vi "ErrorHandler.vi"(5 "user message (\"\")":string, 6 "exception code (0=no exception)":i32, 7 "error description (\"\")":string, 8 "error in (no error)":errorcluster, 11 "error code (0)":i32 format="%0.0f") -> (0 "error out":errorcluster, 2 "Error info":T1)   [LabVIEW 2013, in "SMP.lvclass"]
doc: "Produces an error cluster with a source string that contains all error details in a JSON object. The elements of the JSON object are: Code, Source, Description, Call chain, User message.\n\nThe Description contains the actual/possible cause of the error. This is the standard description that Labview shows when debugging. The \"error in\" input has first priority, so if an error is present here it will be output in \"error out\" with the formatted source string.\n\n<b>error code: </b>If \"error in\" has no error then a custom error will be generated if this code is not 0. The source string of the custom error will have this code, the description from the \"error description\" input, the user message from the \"user message\" input and the call chain up to the VI calling this Error Handler.\n\n<b>error description: </b>The description for the custom error, to be included in the JSON object held in the error source string.\n\n<b>user message: </b>The user message associated with the custom error, to be included in the JSON object held in the error source string.\n\n<b>exception code: </b> Specifies a particular error code to be ignored. This option only works for errors received via the \"error in\" input. If this code is received, the handler will clear the error.\n\n<b>Error info: </b>A cluster containing all error info. This is provided for convenience. It contains exactly the same information as the JSON object held in the error source string."
uses:
  SMP.lvclass
  70a9a6cd-0d05-4d49-a097-5f9bfbe52c2b.vi
  1c7ce2ab-558f-46e0-889c-9a5a86a7245e.vi
  df1b85dd-af5c-4eb8-b3ac-6a4bf91d912d.vi
  cf7a518e-8a90-4b9b-b245-fd60522d3528.vi
  <vilib>/JDP Science/JSONtext/JSONtext.lvlib
  8e39f65f-b52b-460e-aed2-aa7242cb256d.vi
  9ede7785-e4b7-4a2b-ad65-c3c71cf36ef6.vi
  5dddf332-14d7-45ee-9639-52c0eabf6bef.vi
  e595dffb-a454-4284-baeb-2219d1b7dc43.vi
  e26eb3da-07b3-4e20-90df-f977e2e68984.vi
  <vilib>/Utility/error.llb/DialogType.ctl
  debc1eb8-1280-4e15-8515-044490ebb883.vi
  e2486d55-95a2-4599-8c71-563c50abe2ef.vi
  3d1d037f-df6a-40d9-93cf-b9c414a2865f.vi
  7ecf2d71-b2a8-4580-9142-73392cecd242.vi
  1f3aeea1-64a9-4bcd-a0b4-ffb7e781f43c.vi
  b1e9468c-6006-4e50-9a64-d51c3021ee35.vi
  89762134-3b04-4251-8c1b-3ad095ef116d.vi
  12af56b0-901a-41e5-9ea6-8feb9238e45a.vi
  6ee8f00d-676c-48f5-90a6-41a3b84b36f5.vi
  105fa579-688c-41c6-a4d2-67f13b08f2ab.vi
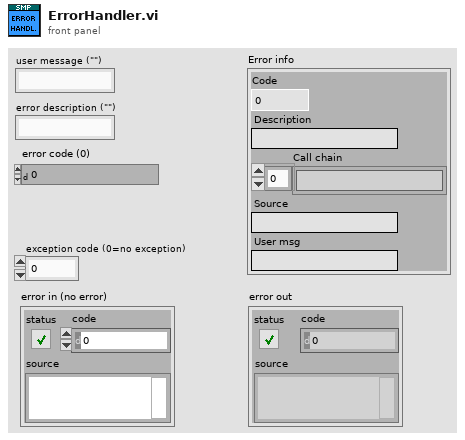
[diagram p1: front panel]
types:
  T1 = cluster{"Code":i32, "Description":string, "Call chain":string[], "Source":string, "User msg":string}
  T2 = typedef "JSONtext.lvlib/JSON Value Type.ctl" = enum16{"Not a JSON Value", "JSON Object", "JSON Array", "String", "Number", "true", "false", "null"}
  T3 = typedef "DialogType.ctl" = u16
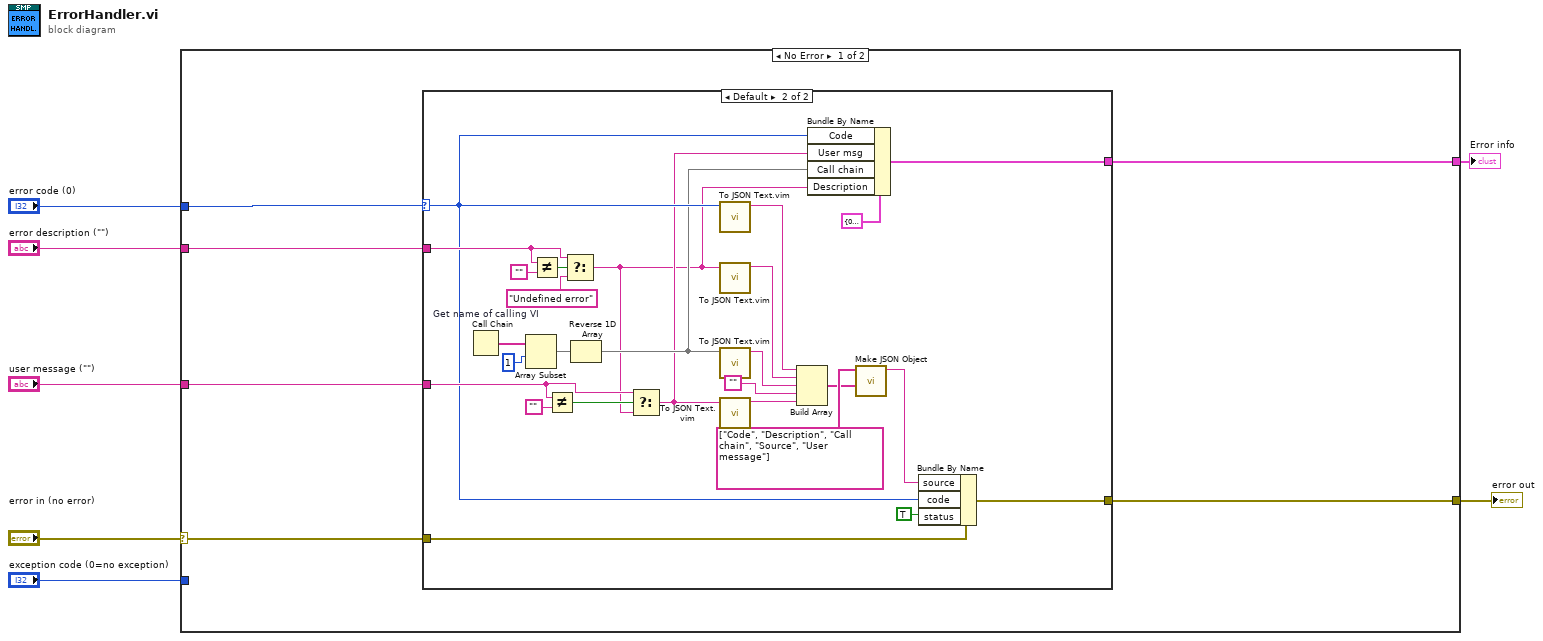
[diagram p0: block diagram]
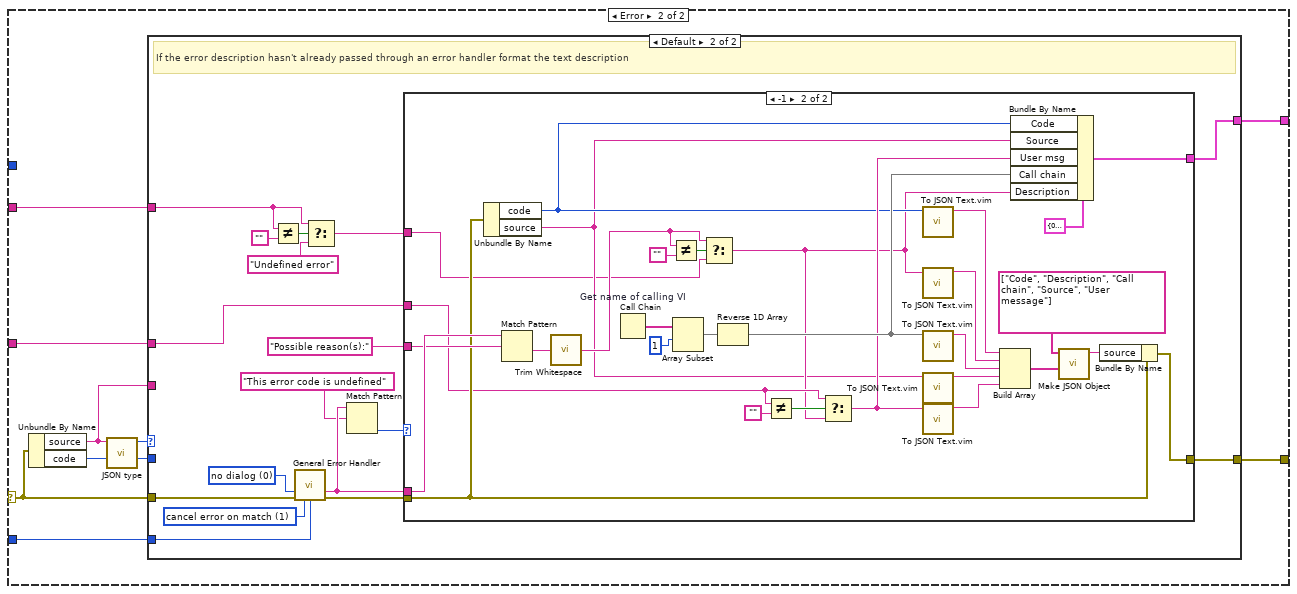
[diagram p3: hidden frame]
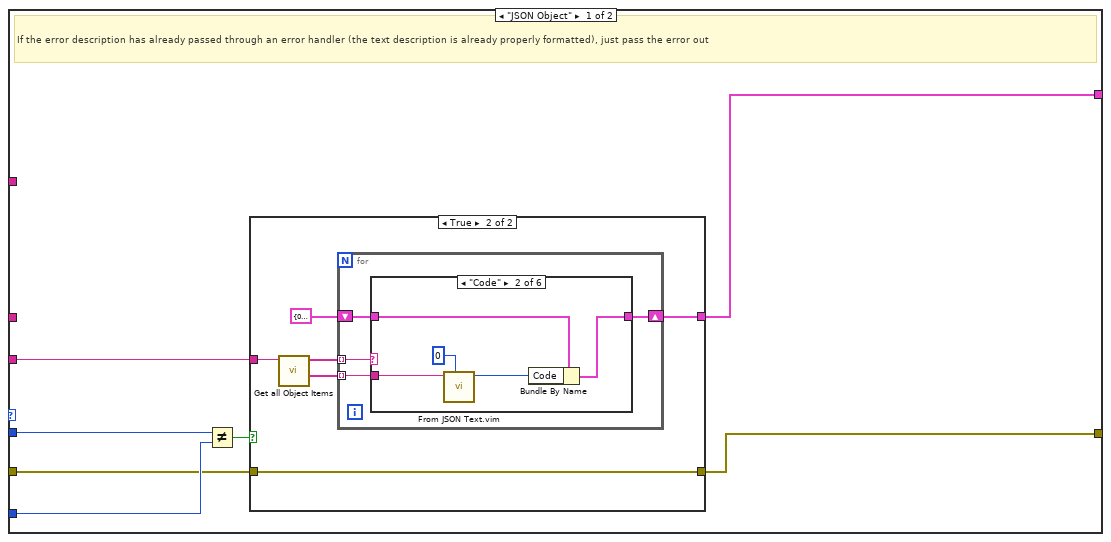
[diagram p4: hidden frame]
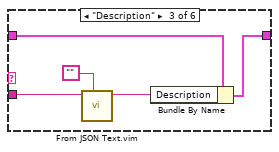
[diagram p7: hidden frame]
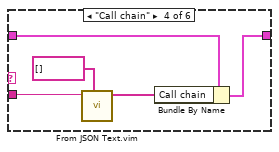
[diagram p8: hidden frame]
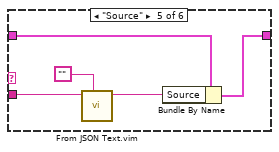
[diagram p9: hidden frame]
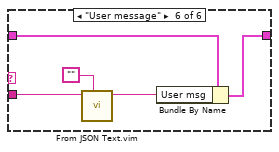
[diagram p10: hidden frame]
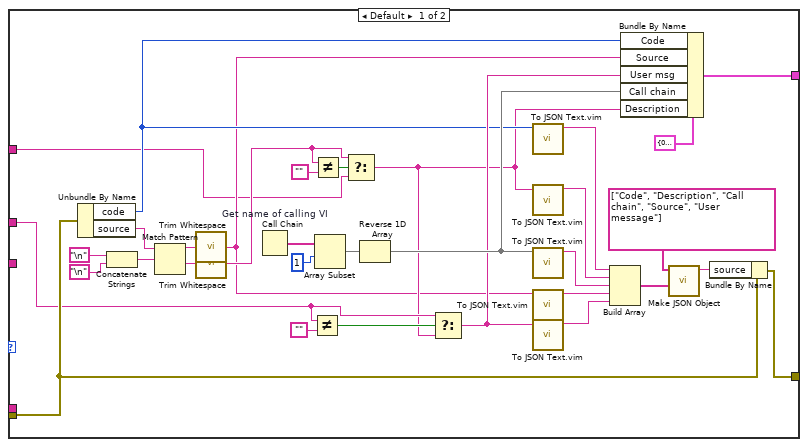
[diagram p11: hidden frame]
diagram:
  n1 = case shown="No Error" "error in (no error)" {
    selector: "error in (no error)" -> [w13 w47]
    tunnel: [w12 w49] -> w7
    tunnel: "error code (0)" -> [w10 _]
    tunnel: "error description (\"\")" -> [w11 w41]
    tunnel: "exception code (0=no exception)" -> [_ w48]
    tunnel: "user message (\"\")" -> [w9 w42]
    tunnel: [w8 w43] -> w1
    frame No Error {
      n2 = case shown="Default" w10 {
        selector: w10 -> [_ w20]
        tunnel: w13 -> [_ w40]
        tunnel: [_ w39] -> w12
        tunnel: w11 -> [_ w35]
        tunnel: w9 -> [_ w28]
        tunnel: [_ w16] -> w8
        frame 0 {
        }
        frame Default {
          n3 = Call Chain "Get name of calling VI"() -> (call chain=w33:string[])
          n4 = Array Subset(array=w33, index=1) -> (w32:string[])  [unwired: 1 in]
          n5 = Not Equal?(x=w35, y="") -> (x != y?=w36:bool)
          n6 = Not Equal?(x=w28, y="") -> (x != y?=w30:bool)
          n7 = Select(t=w35, s=w36, f="Undefined error") -> (s? t:f=w14:string)
          n8 = Reverse 1D Array(array=w32) -> (reversed array=w18:string[])
          n9 = Select(t=w28, s=w30, f=w14) -> (s? t:f=w17:string)
          n10 = call "To JSON Text.vim"("Anything"=w20) -> ("<JSON>"=w25:string)  [unwired: 9 in, 1 out]
          n11 = call "To JSON Text.vim"("Anything"=w14) -> ("<JSON>"=w19:string)  [unwired: 9 in, 1 out]
          n12 = call "To JSON Text.vim"("Anything"=w18) -> ("<JSON>"=w24:string)  [unwired: 9 in, 1 out]
          n13 = call "To JSON Text.vim"("Anything"=w17) -> ("<JSON>"=w23:string)  [unwired: 9 in, 1 out]
          n14 = Build Array(w25, w19, w24, "", w23) -> (w26:string[])
          n15 = Bundle By Name(cluster=T1 {"Code"=0, "Description"="", "Call chain"=[], "Source"="", "User msg"=""}, "Code"=w20, "User msg"=w17, "Call chain"=w18, "Description"=w14) -> (w16:T1)
          n16 = call <vilib>:"Make JSON Object.vi"("JSON Items"=w26, "Item Names"=string[] ["Code", "Description", "Call chain", "Source", "User message"]) -> ("<JSON>"=w22:string)  [unwired: 8 in, 1 out]
          n17 = Bundle By Name(cluster=w40, "source"=w22, "code"=w20, "status"=TRUE) -> (w39:errorcluster)
        }
      }
    }
    frame Error {
      n18 = Unbundle By Name(w47) -> ("source"=w45:string, "code"=w44:i32)
      n19 = call <vilib>:"JSON type.vi"("JSON"=w45) -> ("JSON Value Type"=w46:T2)  [unwired: 9 in, 1 out]
      n20 = case shown="Default" w46 {
        tunnel: [w52 w109] -> w49
        tunnel: w48 -> [w56 w108]
        tunnel: w47 -> [w53 w107]
        tunnel: w45 -> [w55 _]
        tunnel: w44 -> [w54 _]
        tunnel: [w50 w98] -> w43
        tunnel: w42 -> [_ w99]
        tunnel: w41 -> [_ w94]
        frame "JSON Object" {
          # "If the error description has already passed through an error handler (the text description is already properly formatted), just pass the error out"
          n21 = Not Equal?(x=w54, y=w56) -> (x != y?=w51:bool)
          n22 = case shown="True" w51 {
            tunnel: w55 -> [_ w62]
            tunnel: w53 -> [_ w58]
            tunnel: [_ w58] -> w52
            tunnel: [_ w57] -> w50
            frame False {
            }
            frame True {
              n23 = call <vilib>:"Get all Object Items.vi"("JSON"=w62) -> ("<JSON>"=w60:string[], "Item Names"=w61:string[])  [unwired: 7 in, 2 out]
              n24 = for {
                tunnel: w61 -> [w66] mode=indexing
                tunnel: w60 -> [w65] mode=indexing
                shift-right: [w63] -> w57
                shift-left: T1 {"Code"=0, "Description"="", "Call chain"=[], "Source"="", "User msg"=""} -> [w64]
                n25 = case shown="\"Code\"" w66 {
                  tunnel: w65 -> [_ w70 w75 w80 w85 w90]
                  tunnel: w64 -> [w67 w72 w77 w82 w87 w92]
                  tunnel: [w67 w71 w76 w81 w86 w91] -> w63
                  frame Default {
                  }
                  frame "Code" {
                    n26 = call "From JSON Text.vim"("Data Type and Default Value"=0, "JSON"=w70) -> ("Data out"=w68:i32)  [unwired: 8 in, 1 out]
                    n27 = Bundle By Name(cluster=w72, "Code"=w68) -> (w71:T1)
                  }
                  frame "Description" {
                    n28 = call "From JSON Text.vim"("Data Type and Default Value"="", "JSON"=w75) -> ("Data out"=w74:string)  [unwired: 8 in, 1 out]
                    n29 = Bundle By Name(cluster=w77, "Description"=w74) -> (w76:T1)
                  }
                  frame "Call chain" {
                    n30 = call "From JSON Text.vim"("Data Type and Default Value"=string[] [], "JSON"=w80) -> ("Data out"=w79:string[])  [unwired: 8 in, 1 out]
                    n31 = Bundle By Name(cluster=w82, "Call chain"=w79) -> (w81:T1)
                  }
                  frame "Source" {
                    n32 = call "From JSON Text.vim"("Data Type and Default Value"="", "JSON"=w85) -> ("Data out"=w84:string)  [unwired: 8 in, 1 out]
                    n33 = Bundle By Name(cluster=w87, "Source"=w84) -> (w86:T1)
                  }
                  frame "User message" {
                    n34 = call "From JSON Text.vim"("Data Type and Default Value"="", "JSON"=w90) -> ("Data out"=w89:string)  [unwired: 8 in, 1 out]
                    n35 = Bundle By Name(cluster=w92, "User msg"=w89) -> (w91:T1)
                  }
                }
              }
            }
          }
        }
        frame Default {
          w100 = T3 0 items=["no dialog", "OK message", "continue or stop message", "OK message + warnings", "continue/stop + warnings"] ("type of dialog (OK msg:1)")
          w105 = 1 items=["no exception", "cancel error on match", "set error on match"] ("[exception action] (none:0)")
          # "If the error description hasn't already passed through an error handler format the text description"
          n36 = Not Equal?(x=w94, y="") -> (x != y?=w95:bool)
          n37 = call <vilib>:"General Error Handler.vi"("type of dialog (OK msg:1)"=w100, "error in (no error)"=w107, "[exception action] (none:0)"=w105, "[exception code]"=w108) -> ("message"=w104:string, "error out"=w106:errorcluster)  [unwired: 7 in, 3 out]
          n38 = Select(t=w94, s=w95, f="Undefined error") -> (s? t:f=w93:string)
          n39 = Match Pattern(string=w104, regular expression="This error code is undefined") -> (offset past match=w102:i32)  [unwired: 1 in, 3 out]
          n40 = case shown="-1" w102 {
            tunnel: [w116 w152] -> w109
            tunnel: w106 -> [w142 w149]
            tunnel: w104 -> [_ w172]
            tunnel: "Possible reason(s):" ("search string") -> [_ w171]
            tunnel: w99 -> [w117 w147]
            tunnel: [w114 w151] -> w98
            tunnel: w93 -> [w110 w143]
            frame Default {
              n41 = Unbundle By Name(w142) -> ("code"=w119:i32, "source"=w138:string)
              n42 = Concatenate Strings("\n", "\n") -> (w139:string)
              n43 = Match Pattern(string=w138, regular expression=w139) -> (before substring=w137:string, after substring=w136:string)  [unwired: 1 in, 2 out]
              n44 = call <vilib>:"Trim Whitespace.vi"("string"=w137) -> ("trimmed string"=w111:string)  [unwired: 1 in]
              n45 = call <vilib>:"Trim Whitespace.vi"("string"=w136) -> ("trimmed string"=w118:string)  [unwired: 1 in]
              n46 = Call Chain "Get name of calling VI"() -> (call chain=w134:string[])
              n47 = Not Equal?(x=w117, y="") -> (x != y?=w132:bool)
              n48 = Not Equal?(x=w118, y="") -> (x != y?=w135:bool)
              n49 = Array Subset(array=w134, index=1) -> (w133:string[])  [unwired: 1 in]
              n50 = Select(t=w118, s=w135, f=w110) -> (s? t:f=w113:string)
              n51 = Reverse 1D Array(array=w133) -> (reversed array=w126:string[])
              n52 = Select(t=w117, s=w132, f=w113) -> (s? t:f=w125:string)
              n53 = call "To JSON Text.vim"("Anything"=w119) -> ("<JSON>"=w130:string)  [unwired: 9 in, 1 out]
              n54 = call "To JSON Text.vim"("Anything"=w113) -> ("<JSON>"=w127:string)  [unwired: 9 in, 1 out]
              n55 = call "To JSON Text.vim"("Anything"=w126) -> ("<JSON>"=w129:string)  [unwired: 9 in, 1 out]
              n56 = call "To JSON Text.vim"("Anything"=w111) -> ("<JSON>"=w112:string)  [unwired: 9 in, 1 out]
              n57 = call "To JSON Text.vim"("Anything"=w125) -> ("<JSON>"=w128:string)  [unwired: 9 in, 1 out]
              n58 = Build Array(w130, w127, w129, w112, w128) -> (w131:string[])
              n59 = Bundle By Name(cluster=T1 {"Code"=0, "Description"="", "Call chain"=[], "Source"="", "User msg"=""}, "Code"=w119, "Source"=w111, "User msg"=w125, "Call chain"=w126, "Description"=w113) -> (w114:T1)
              n60 = call <vilib>:"Make JSON Object.vi"("JSON Items"=w131, "Item Names"=string[] ["Code", "Description", "Call chain", "Source", "User message"]) -> ("<JSON>"=w115:string)  [unwired: 8 in, 1 out]
              n61 = Bundle By Name(cluster=w142, "source"=w115) -> (w116:errorcluster)
            }
            frame -1 {
              n62 = Unbundle By Name(w149) -> ("code"=w148:i32, "source"=w144:string)
              n63 = Match Pattern(string=w172, regular expression=w171) -> (after substring=w170:string)  [unwired: 1 in, 3 out]
              n64 = call <vilib>:"Trim Whitespace.vi"("string"=w170) -> ("trimmed string"=w150:string)  [unwired: 1 in]
              n65 = Call Chain "Get name of calling VI"() -> (call chain=w168:string[])
              n66 = Not Equal?(x=w150, y="") -> (x != y?=w169:bool)
              n67 = Array Subset(array=w168, index=1) -> (w167:string[])  [unwired: 1 in]
              n68 = Select(t=w150, s=w169, f=w143) -> (s? t:f=w146:string)
              n69 = Reverse 1D Array(array=w167) -> (reversed array=w160:string[])
              n70 = Not Equal?(x=w147, y="") -> (x != y?=w166:bool)
              n71 = Select(t=w147, s=w166, f=w146) -> (s? t:f=w159:string)
              n72 = call "To JSON Text.vim"("Anything"=w148) -> ("<JSON>"=w164:string)  [unwired: 9 in, 1 out]
              n73 = call "To JSON Text.vim"("Anything"=w146) -> ("<JSON>"=w161:string)  [unwired: 9 in, 1 out]
              n74 = call "To JSON Text.vim"("Anything"=w160) -> ("<JSON>"=w163:string)  [unwired: 9 in, 1 out]
              n75 = call "To JSON Text.vim"("Anything"=w144) -> ("<JSON>"=w145:string)  [unwired: 9 in, 1 out]
              n76 = call "To JSON Text.vim"("Anything"=w159) -> ("<JSON>"=w162:string)  [unwired: 9 in, 1 out]
              n77 = Build Array(w164, w161, w163, w145, w162) -> (w165:string[])
              n78 = Bundle By Name(cluster=T1 {"Code"=0, "Description"="", "Call chain"=[], "Source"="", "User msg"=""}, "Code"=w148, "Source"=w144, "User msg"=w159, "Call chain"=w160, "Description"=w146) -> (w151:T1)
              n79 = call <vilib>:"Make JSON Object.vi"("JSON Items"=w165, "Item Names"=string[] ["Code", "Description", "Call chain", "Source", "User message"]) -> ("<JSON>"=w158:string)  [unwired: 8 in, 1 out]
              n80 = Bundle By Name(cluster=w149, "source"=w158) -> (w152:errorcluster)
            }
          }
        }
      }
    }
  }
  "error out" <- w7
  "Error info" <- w1
